vi "ScanAction.vi"(8 "error in (no error)":errorcluster caption="entrée d'erreur (pas d'erreur)", 9 "IndicePoint":i32, 10 "Dir":bool, 11 "Tools In":refnum<class "E8267D.lvclass"> caption="DNL_LabVIEW Object in") -> (0 "error out":errorcluster caption="sortie d'erreur", 2 "ScanParsOut":dbl[](array[numeric]), 3 "Tools Out":refnum<class "E8267D.lvclass"> caption="DNL_LabVIEW Object out")   [LabVIEW 2019, in "E8267D.lvclass"]
uses:
  E8267D.lvclass
  C:/Programmes Labview/LabscanV1A/DevicesClass/BaseDevice/BaseDevice.lvclass
  E8267D.lvclass/E8267D.ctl
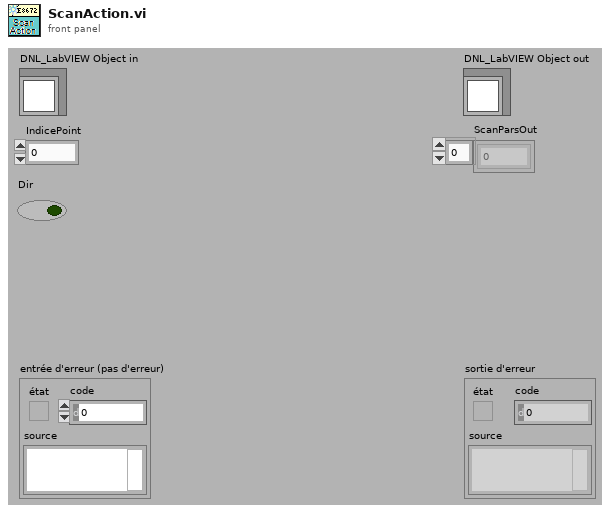
[diagram p1: front panel]
types:
  T1 = typedef "E8267D.lvclass/E8267D_Func.ctl" = enum16{"SetPower (dBm)", "SetFrequency (Hz)"}
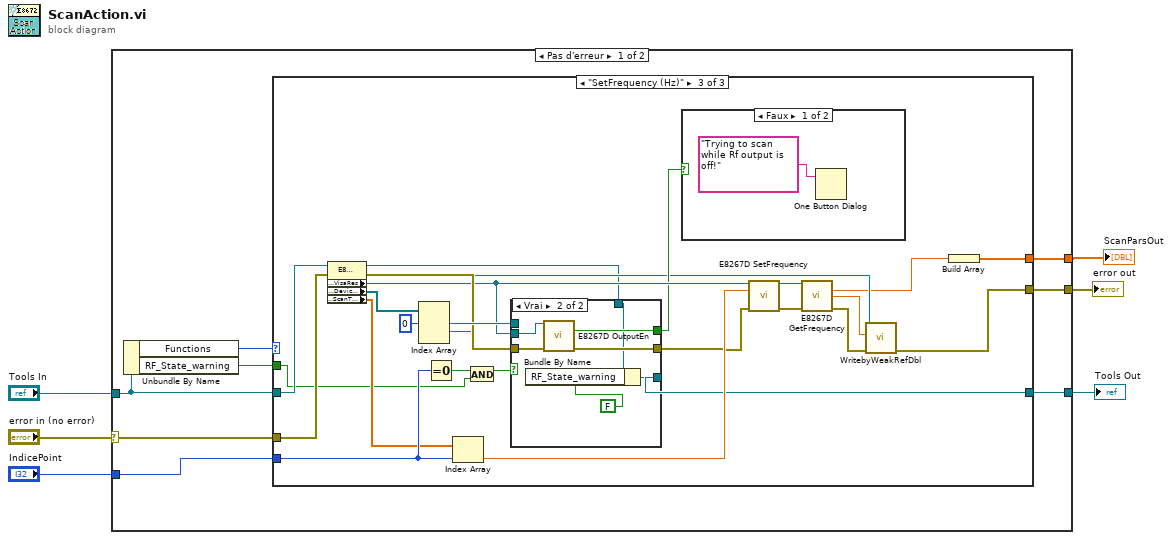
[diagram p0: block diagram]
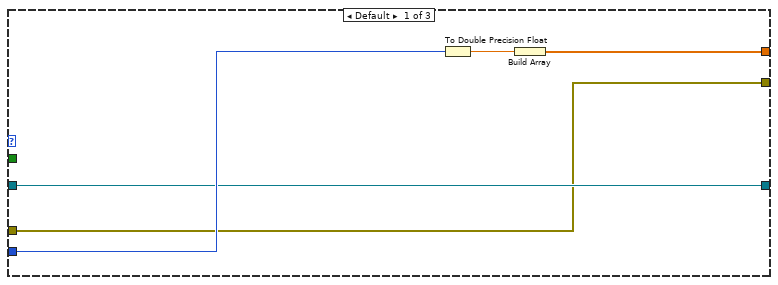
[diagram p2: hidden frame]
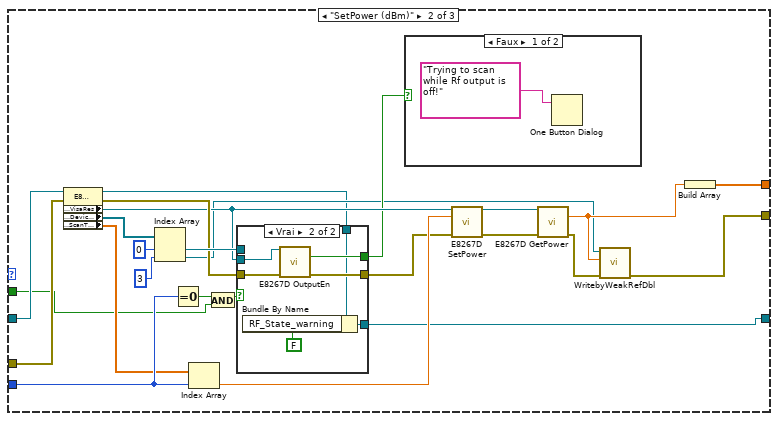
[diagram p3: hidden frame]
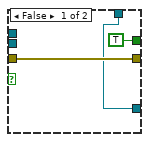
[diagram p5: hidden frame]
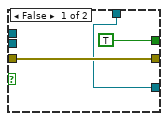
[diagram p7: hidden frame]
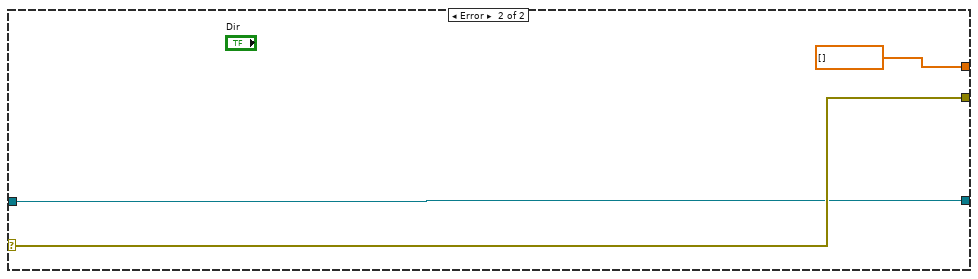
[diagram p8: hidden frame]
diagram:
  n1 = case shown="Pas d'erreur" "error in (no error)" {
    selector: "error in (no error)" -> [w11 w94]
    tunnel: "Tools In" -> [w12 w93]
    tunnel: [w10 dbl[] []] -> w1
    tunnel: [w9 w94] -> w4
    tunnel: [w8 w93] -> w3
    tunnel: "IndicePoint" -> [w13 _]
    frame No Error {
      n2 = Unbundle By Name(w12) -> ("Functions"=w14:T1, "RF_State_warning"=w7:bool)
      n3 = case shown="\"SetFrequency (Hz)\"" w14 {
        tunnel: [w15 w39 w75] -> w10
        tunnel: w13 -> [w19 w31 w69]
        tunnel: [w17 w20 w56] -> w8
        tunnel: w12 -> [w17 w36 w73]
        tunnel: w11 -> [w16 w42 w78]
        tunnel: [w16 w25 w65] -> w9
        tunnel: w7 -> [_ w22 w58]
        frame Default {
          n4 = To Double Precision Float(number=w19) -> (double precision float=w18:dbl)
          n5 = Build Array(w18) -> (w15:dbl[])
        }
        frame "SetPower (dBm)" {
          n6 = property class="E8267D.lvclass"(reference=w36, error in=w42) -> (reference out=w21:refnum<class "E8267D.lvclass">, error out=w34:errorcluster, "Accessor:VisaRes"=w30:refnum<visa-resource-name>, "Accessor:DeviceCtrl"=w40:refnum<vi>[], "Accessor:ScanTable"=w24:dbl[])
          n7 = Index Array(array=w40, index #1=0 ("indice"), index #2=3 ("indice")) -> (element #1=w35:refnum<vi>, element #2=w26:refnum<vi>)
          n8 = Equal To 0?(x=w31) -> (x = 0?=w32:bool)
          n9 = Index Array(array=w24, index=w31) -> (element=w41:dbl)
          n10 = And(x=w32, y=w22) -> (x .and. y?=w23:bool)
          n11 = case shown="Vrai" w23 {
            tunnel: w35 -> [_ _]
            tunnel: w34 -> [w48 w54]
            tunnel: [w48 w53] -> w33
            tunnel: w30 -> [_ w55]
            tunnel: [TRUE ("Enabled") w52] -> w29
            tunnel: w21 -> [w46 w51]
            tunnel: [w46 w49] -> w20
            frame False {
            }
            frame True {
              n12 = Bundle By Name(cluster=w51, "RF_State_warning"=FALSE) -> (w49:refnum<class "E8267D.lvclass">)
              n13 = call <userlib>:"E8267D OutputEn.vi"("VISA Rsrc"=w55, "error in (no error)"=w54) -> ("Enabled"=w52:bool, "error out"=w53:errorcluster)  [unwired: 11 in, 1 out]
            }
          }
          n14 = case shown="Faux" w29 {
            frame False {
              n15 = One Button Dialog(message="Trying to scan while Rf output is off!") -> ()  [unwired: 1 in, 1 out]
            }
            frame True {
            }
          }
          n16 = call <userlib>:"E8267D SetPower.vi"("VISA Rsrc"=w30, "Power dBm"=w41, "error in (no error)"=w33) -> ("VISA Rsrc Out"=w43:refnum<visa-resource-name>, "error out"=w44:errorcluster)  [unwired: 11 in]
          n17 = call <userlib>:"E8267D GetPower.vi"("VISA Rsrc"=w43, "error in (no error)"=w44) -> ("Power (dBm)"=w27:dbl, "error out"=w28:errorcluster)  [unwired: 11 in, 1 out]
          n18 = call <userlib>:"WritebyWeakRefDbl.vi"("error in"=w28, "Valeur"=w27, "Control Ref"=w26) -> ("error out"=w25:errorcluster)  [unwired: 8 in]
          n19 = Build Array(w27) -> (w39:dbl[])
        }
        frame "SetFrequency (Hz)" {
          n20 = property class="E8267D.lvclass"(reference=w73, error in=w78) -> (reference out=w57:refnum<class "E8267D.lvclass">, error out=w71:errorcluster, "Accessor:VisaRes"=w68:refnum<visa-resource-name>, "Accessor:DeviceCtrl"=w76:refnum<vi>[], "Accessor:ScanTable"=w62:dbl[])
          n21 = Index Array(array=w76, index #1=0 ("indice")) -> (element #1=w72:refnum<vi>, element #2=w64:refnum<vi>)  [unwired: 2 in, 1 out]
          n22 = Equal To 0?(x=w69) -> (x = 0?=w70:bool)
          n23 = Index Array(array=w62, index=w69) -> (element=w77:dbl)
          n24 = And(x=w70, y=w58) -> (x .and. y?=w59:bool)
          n25 = case shown="Vrai" w59 {
            tunnel: w72 -> [_ _]
            tunnel: w71 -> [w84 w90]
            tunnel: [w84 w89] -> w60
            tunnel: w68 -> [_ w91]
            tunnel: [TRUE ("Enabled") w88] -> w67
            tunnel: w57 -> [w82 w87]
            tunnel: [w82 w85] -> w56
            frame False {
            }
            frame True {
              n26 = Bundle By Name(cluster=w87, "RF_State_warning"=FALSE) -> (w85:refnum<class "E8267D.lvclass">)
              n27 = call <userlib>:"E8267D OutputEn.vi"("VISA Rsrc"=w91, "error in (no error)"=w90) -> ("Enabled"=w88:bool, "error out"=w89:errorcluster)  [unwired: 11 in, 1 out]
            }
          }
          n28 = case shown="Faux" w67 {
            frame False {
              n29 = One Button Dialog(message="Trying to scan while Rf output is off!") -> ()  [unwired: 1 in, 1 out]
            }
            frame True {
            }
          }
          n30 = call <userlib>:"E8267D SetFrequency.vi"("VISA Rsrc"=w68, "Frequency (Hz)"=w77, "error in (no error)"=w60) -> ("VISA Rsrc Out"=w79:refnum<visa-resource-name>, "error out"=w80:errorcluster)  [unwired: 11 in]
          n31 = call <userlib>:"E8267D GetFrequency.vi"("VISA Rsrc"=w79, "error in (no error)"=w80) -> ("Frequency (Hz)"=w61:dbl, "Frequency (Units)"=w63:dbl, "error out"=w66:errorcluster)  [unwired: 10 in, 1 out]
          n32 = call <userlib>:"WritebyWeakRefDbl.vi"("error in"=w66, "Valeur"=w63, "Control Ref"=w64) -> ("error out"=w65:errorcluster)  [unwired: 8 in]
          n33 = Build Array(w61) -> (w75:dbl[])
        }
      }
    }
    frame Error {
    }
  }
  "error out" <- w4
  "Tools Out" <- w3
  "ScanParsOut" <- w1
